vi "PicoScope6000GetValues.vi"(5 "Segment Range":T1 {"toSegmentIndex" format="%.4p"; "fromSegmentIndex" format="%.4p"}, 7 "Buffer and Transfer Settings":T2 {"Down-Sample Mode" items=["RAW none", "None", "Aggregate", "Decimate", "Average"]; "Down Sample Ratio" step=1; "Samples" format="%_6p"}, 8 "error in (no error)":errorcluster, 11 "handle in":i16) -> (0 "error out":errorcluster, 3 "handle out":i16, 4 "overflow":i16 format="%010b", 6 "noOfSamples":u64)   [LabVIEW 2009]
doc: "Calls ps5000aGetValuesOverlapped"
uses:
  ps6000.dll
  shared/Buffer and Transfer Settings.ctl
  shared/Segment Range.ctl
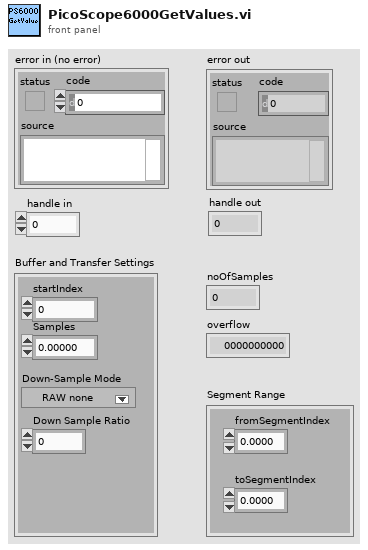
[diagram p1: front panel]
types:
  T1 = typedef "Segment Range.ctl" = cluster{"fromSegmentIndex":u64, "toSegmentIndex":u64}
  T2 = typedef "Buffer and Transfer Settings.ctl" = cluster{"startIndex":u64, "Samples":u64, "Down Sample Ratio":u64, "Down-Sample Mode":u32}
  T3 = cluster{"status":bool, "code":u32, "source":string}
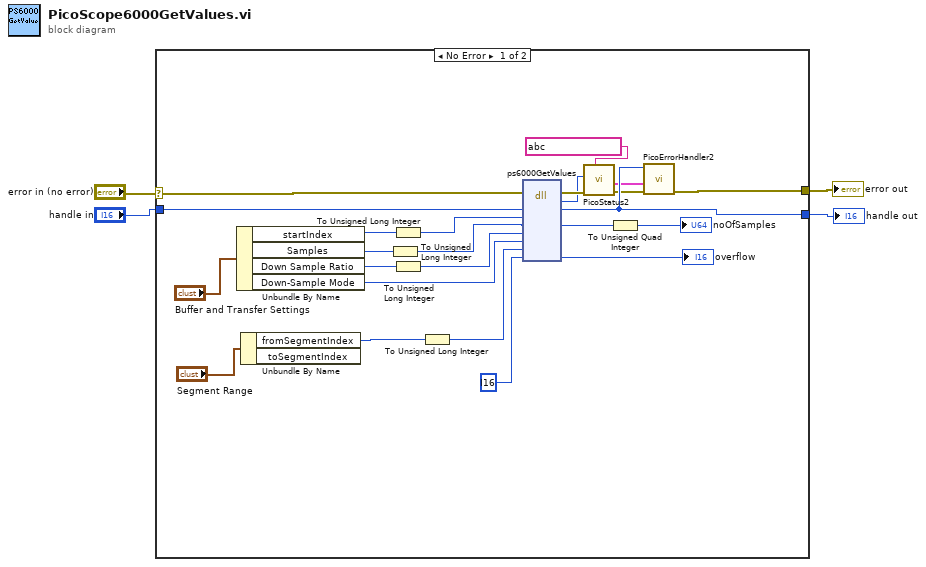
[diagram p0: block diagram]
diagram:
  n1 = case shown="No Error" "error in (no error)" {
    selector: "error in (no error)" -> [w26 w29]
    tunnel: "handle in" -> [w25 w30]
    tunnel: [w12 w30] -> w4
    tunnel: [w24 w29] -> w3
    frame #0 {
      n2 = Unbundle By Name("Buffer and Transfer Settings") -> ("startIndex"=w19:u64, "Samples"=w17:u64, "Down Sample Ratio"=w18:u64, "Down-Sample Mode"=w13:u32)
      n3 = Unbundle By Name("Segment Range") -> ("fromSegmentIndex"=w21:u64)  [unwired: 1 out]
      n4 = To Unsigned Long Integer(number=w17) -> (unsigned 32bit integer=w15:u32)
      n5 = To Unsigned Long Integer(number=w19) -> (unsigned 32bit integer=w16:u32)
      n6 = To Unsigned Long Integer(number=w18) -> (unsigned 32bit integer=w14:u32)
      n7 = To Unsigned Long Integer(number=w21) -> (unsigned 32bit integer=w20:u32)
      n8 = dll-call lib="ps6000.dll" fn="ps6000GetValues" ("ps3000.dll:_ps3000_open_unit@0")(error in=w26, "handle"=w25, "startIndex"=w16, "noOfSamples"=w15, "downSampleRatio"=w14, "downSampleRatioMode"=w13, "segmentIndex"=w20, "overflow"=i16 ?) -> (error out=w8:errorcluster, "PICO_STATUS"=w7:u32, "handle"=w12:i16, "noOfSamples"=w11:u32, "overflow"=→"overflow":i16)  [unwired: 6 in, 1 out]
      n9 = call "PicoStatus2.vi"("PICO source"=string ? ("source"), "Error in"=w8, "PICO STATUS"=w7) -> ("error out"=w9:errorcluster, "PICO_STATUS out"=w5:T3)  [unwired: 5 in]
      n10 = To Unsigned Quad Integer(1:w11) -> (0:→"noOfSamples":u64)
      n11 = call "PicoErrorHandler2.vi"("error in (no error)"=w9, "PICO_STATUS in"=w5, "handle In"=w12) -> ("error out"=w24:errorcluster)  [unwired: 8 in]
    }
    frame #1 {
    }
  }
  "error out" <- w3
  "handle out" <- w4
